vi "FPGA_controller.vi"() -> ()   [LabVIEW 2017]
uses:
  <vilib>/rvi/Emulation/niFpgaGetClockAttributes.vi
  <vilib>/rvi/Emulation/niFpgaSctlEmulationGetInTimedLoop.vi
  <vilib>/rvi/Emulation/niFpgaEmulationReportErrorSimple.vi
  <vilib>/rvi/eio/common/nirviEmuTemplateMethod_errors.vi
  <vilib>/rvi/Emulation/niFpgaCriticalErrorInLSC.vi
  <vilib>/eio/EIONode/EIONode.xnode
panel:
  in  "Scale x2":fxp<+/-,32,16>=10.0 format="%#_21g"
  in  "m_first x2":fxp<+/-,49,33>=4.9499969482421875 format="%#_26g"
  in  "Offset x2":fxp<+/-,48,32> format="%#_26g"
  in  "1/eta x":fxp<+/-,32,16>=200.0 format="%#_21g"
  in  "m_first x1":fxp<+/-,49,33>=0.649993896484375 format="%#_26g"
  in  "Offset x1":fxp<+/-,48,32> format="%#_26g"
  in  "Scale x1":fxp<+/-,32,16>=5.0 format="%#_21g"
  in  "stop 2":bool
  # "STATES CONVERSION"
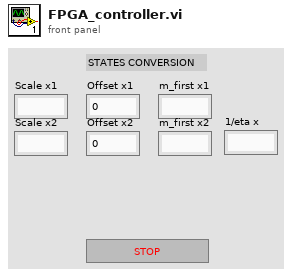
[diagram p1: front panel]
types:
  T1 = cluster{"Boolean array[0]":bool, "Boolean array[1]":bool, "Boolean array[2]":bool, "Boolean array[3]":bool, "Boolean array[4]":bool, "Boolean array[5]":bool, "Boolean array[6]":bool, "Boolean array[7]":bool, "Boolean array[8]":bool, "Boolean array[9]":bool, "Boolean array[10]":bool, "Boolean array[11]":bool, "Boolean array[12]":bool, "Boolean array[13]":bool, "Boolean array[14]":bool, "Boolean array[15]":bool}
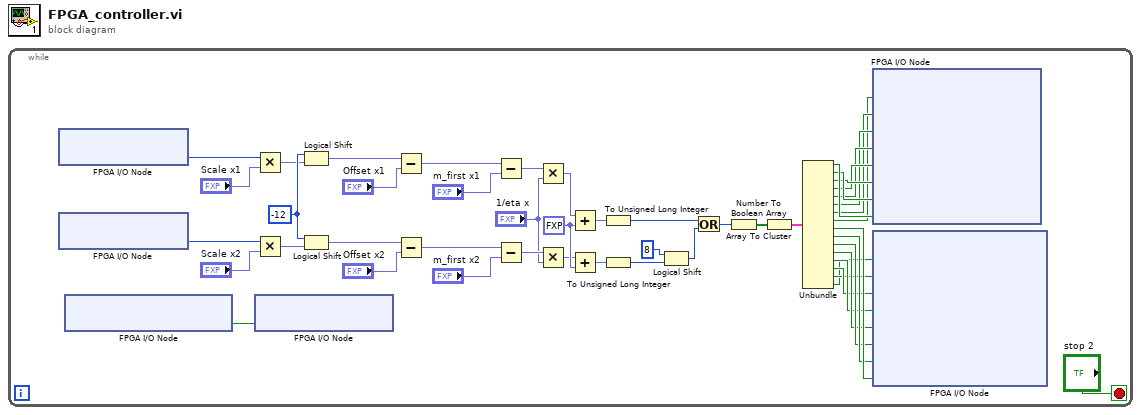
[diagram p0: block diagram]
diagram:
  n1 = while {
    stop <- "stop 2" stop-if-true
    w24 = fxp<+/-,64,32> 0.5 ("y")
    w22 = i16 -12 ("y")
    n2 = xnode "FPGA I/O Node"() -> ("ConnectorA/AI0"=w9:u16)  [unwired: 1 in, 1 out]
    n3 = xnode "FPGA I/O Node"() -> ("ConnectorA/AI1"=w7:u16)  [unwired: 1 in, 1 out]
    n4 = xnode "FPGA I/O Node"() -> ("Component-Level IP\\f0"=w31:bool)  [unwired: 1 in, 1 out]
    n5 = Multiply(x=w9, y="Scale x1") -> (x*y=w21:fxp<+/-,48,32>)
    n6 = Multiply(x=w7, y="Scale x2") -> (x*y=w25:fxp<+/-,48,32>)
    n7 = xnode "FPGA I/O Node"("ConnectorA/DIO0"=w31) -> ()  [unwired: 1 in, 1 out]
    n8 = Logical Shift(y=w22, x=w21) -> (x << y=w18:fxp<+/-,48,32>)
    n9 = Logical Shift(y=w22, x=w25) -> (x << y=w15:fxp<+/-,48,32>)
    n10 = Subtract(x=w18, y="Offset x1") -> (x-y=w19:fxp<+/-,49,33>)
    n11 = Subtract(x=w15, y="Offset x2") -> (x-y=w16:fxp<+/-,49,33>)
    n12 = Subtract(x=w19, y="m_first x1") -> (x-y=w20:fxp<+/-,50,34>)
    n13 = Subtract(x=w16, y="m_first x2") -> (x-y=w14:fxp<+/-,50,34>)
    n14 = Multiply(x=w20, y="1/eta x") -> (x*y=w17:fxp<+/-,64,49>)
    n15 = Multiply(x=w14, y="1/eta x") -> (x*y=w13:fxp<+/-,64,49>)
    n16 = Add(x=w17, y=w24) -> (x+y=w30:fxp<+/-,64,50>)
    n17 = Add(x=w13, y=w24) -> (x+y=w23:fxp<+/-,64,50>)
    n18 = To Unsigned Long Integer(number=w30) -> (unsigned 32bit integer=w26:u32)
    n19 = To Unsigned Long Integer(number=w23) -> (unsigned 32bit integer=w28:u32)
    n20 = Logical Shift(y=8, x=w28) -> (x << y=w27:u32)
    n21 = Or(x=w26, y=w27) -> (x .or. y?=w10:u32)
    n22 = Number To Boolean Array(number=w10) -> (Boolean array=w11:bool[])
    n23 = Array To Cluster(array=w11) -> (cluster=w48:T1)
    n24 = Unbundle(w48) -> ("Boolean array[0]"=w47:bool, "Boolean array[1]"=w46:bool, "Boolean array[2]"=w45:bool, "Boolean array[3]"=w44:bool, "Boolean array[4]"=w43:bool, "Boolean array[5]"=w42:bool, "Boolean array[6]"=w41:bool, "Boolean array[7]"=w40:bool, "Boolean array[8]"=w39:bool, "Boolean array[9]"=w38:bool, "Boolean array[10]"=w37:bool, "Boolean array[11]"=w36:bool, "Boolean array[12]"=w35:bool, "Boolean array[13]"=w34:bool, "Boolean array[14]"=w33:bool, "Boolean array[15]"=w32:bool)
    n25 = xnode "FPGA I/O Node"("Component-Level IP\\x0"=w40, "Component-Level IP\\x1"=w41, "Component-Level IP\\x2"=w42, "Component-Level IP\\x3"=w43, "Component-Level IP\\x4"=w44, "Component-Level IP\\x5"=w45, "Component-Level IP\\x6"=w46, "Component-Level IP\\x7"=w47) -> ()  [unwired: 8 in, 8 out]
    n26 = xnode "FPGA I/O Node"("Component-Level IP\\x8"=w32, "Component-Level IP\\x9"=w33, "Component-Level IP\\x10"=w34, "Component-Level IP\\x11"=w35, "Component-Level IP\\x12"=w36, "Component-Level IP\\x13"=w37, "Component-Level IP\\x14"=w38, "Component-Level IP\\x15"=w39) -> ()  [unwired: 8 in, 8 out]
  }
